vi "Visit Me.vi"(8 "error in (no error)":errorcluster, 10 "Visitor In":refnum<class "LVTypeVisitor.lvclass">, 11 "LVArrayType in":refnum<class "LVArrayType.lvclass">) -> (0 "error out":errorcluster, 2 "Visitor Out":refnum<class "LVTypeVisitor.lvclass">, 3 "LVArrayType out":refnum<class "LVArrayType.lvclass">)   [LabVIEW 2020, in "LVDataTypes.lvlib" / "LVArrayType.lvclass"]
uses:
  <vilib>/AppBuilder/Engine/WebServiceDescription/LVDataTypes/LVArrayType/LVArrayType.lvclass
  <vilib>/AppBuilder/Engine/WebServiceDescription/LVDataTypes/LVTypeVisitor/LVTypeVisitor.lvclass
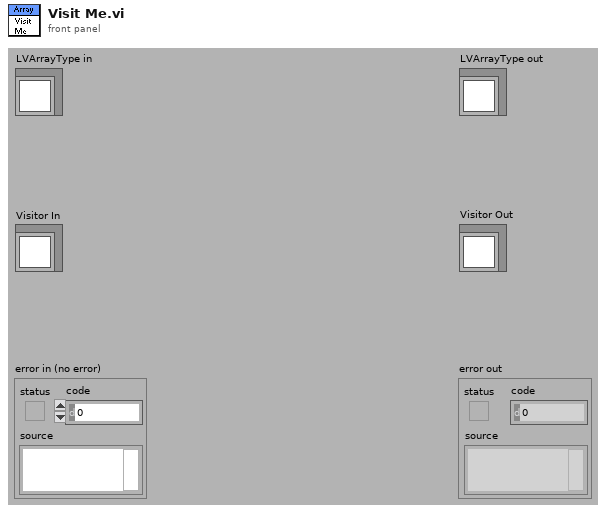
[diagram p1: front panel]
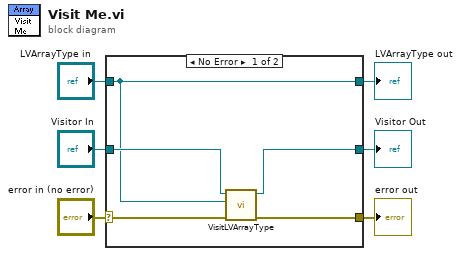
[diagram p0: block diagram]
diagram:
  n1 = case shown="No Error" "error in (no error)" {
    selector: "error in (no error)" -> [w8 w14]
    tunnel: [w7 w14] -> w5
    tunnel: "Visitor In" -> [w11 w13]
    tunnel: [w10 w13] -> w3
    tunnel: "LVArrayType in" -> [w9 w12]
    tunnel: [w9 w12] -> w1
    frame No Error {
      n2 = call-dynamic "VisitLVArrayType.vi"("error in (no error)"=w8, "LVArrayType"=w9, "LVTypeVisitor in"=w11) -> ("error out"=w7:errorcluster, "LVTypeVisitor out"=w10:refnum<class "LVTypeVisitor.lvclass">)  [unwired: 7 out]
    }
    frame Error {
    }
  }
  "error out" <- w5
  "LVArrayType out" <- w1
  "Visitor Out" <- w3
